vi "BarcodeFunc (1).vi"() -> ()   [LabVIEW 2016, in "Team234_Project5.lvrbt"]
uses:
  Team234_Project5.lvrbt
  <vilib>/NXT/Block Support/NXT_InputPort.ctl
  <vilib>/NXT/Subs/ColorSensorColors.ctl
  <vilib>/NXT/Subs/LVHSConnector.ctl
  <vilib>/NXT/LegoClasses/BrickReference/BrickReference.lvclass
  <vilib>/NXT/Block Support/NXT_OutputPort.ctl
  <vilib>/NXT/Dual Mode Library/Sensors/EV3_Color_Color.vi
  <vilib>/NXT/Dual Mode Library/Sound/Tone.vi
  <vilib>/NXT/NXTIO Xnodes/NXTIONodeSubVIs/NXTMoveMotors.vi
  <vilib>/NXT/Dual Mode Library/Waits/Wait_Num.vi
  <vilib>/NXT/NXTIO Xnodes/AddressXNode/NXTIOAddress.xnode
  <vilib>/NXT/NXTIO Xnodes/NXTIOXNode/NXTIO.xnode
panel:
  in  "NXT/EV3":T1
  out "NXT/EV3 10":T1
  in  "Time (1 sec) 3":sgl=1.0
  in  "Power/Speed 6":i8=75
  in  "Power/Speed 5":i8=75
  out "NXT/EV3 9":T1
  in  "Tone (440 Hz) 3":u16=440
  in  "Duration (500 ms) 3":u16=500
  out "Detected Color 2":T2
  in  "Port (Port 1) 2":T3 items=["Port 1", "Port 2", "Port 3", "Port 4"]
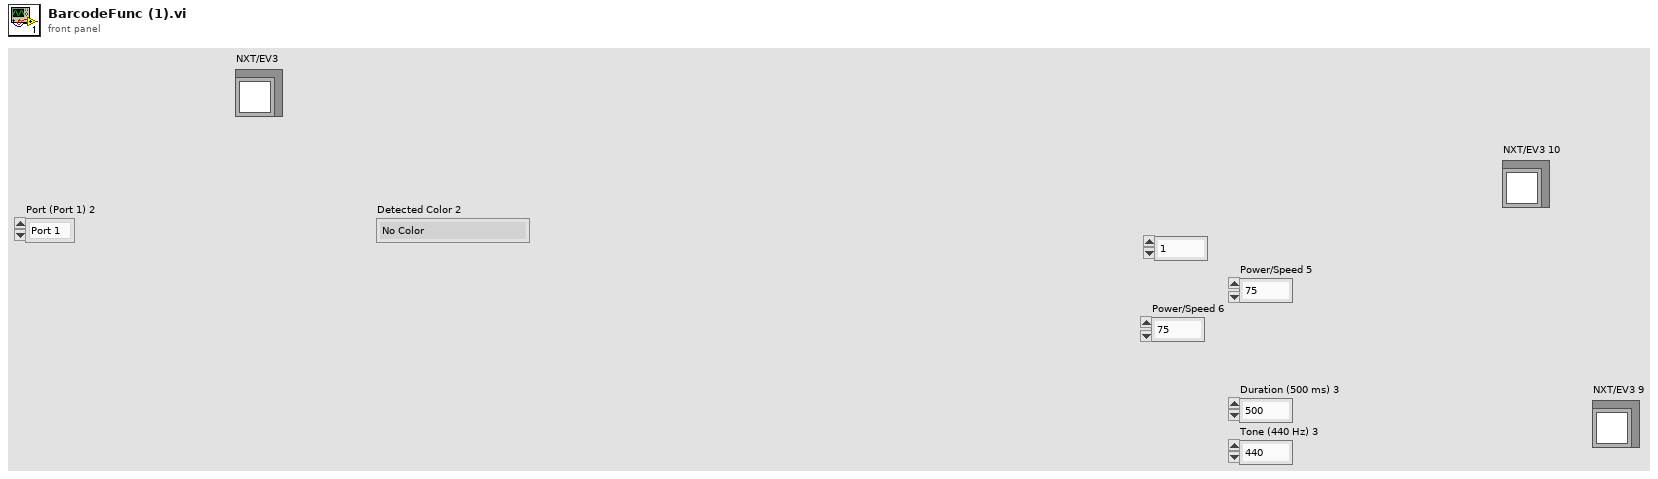
[diagram p1: front panel]
types:
  T1 = typedef "LVHSConnector.ctl" = refnum<class "BrickReference.lvclass">
  T2 = typedef "ColorSensorColors.ctl" = enum16{"No Color", "Black", "Blue", "Green", "Yellow", "Red", "White", "Brown"}
  T3 = typedef "NXT_InputPort.ctl" = u32
  T4 = typedef "NXT_OutputPort.ctl" = u8
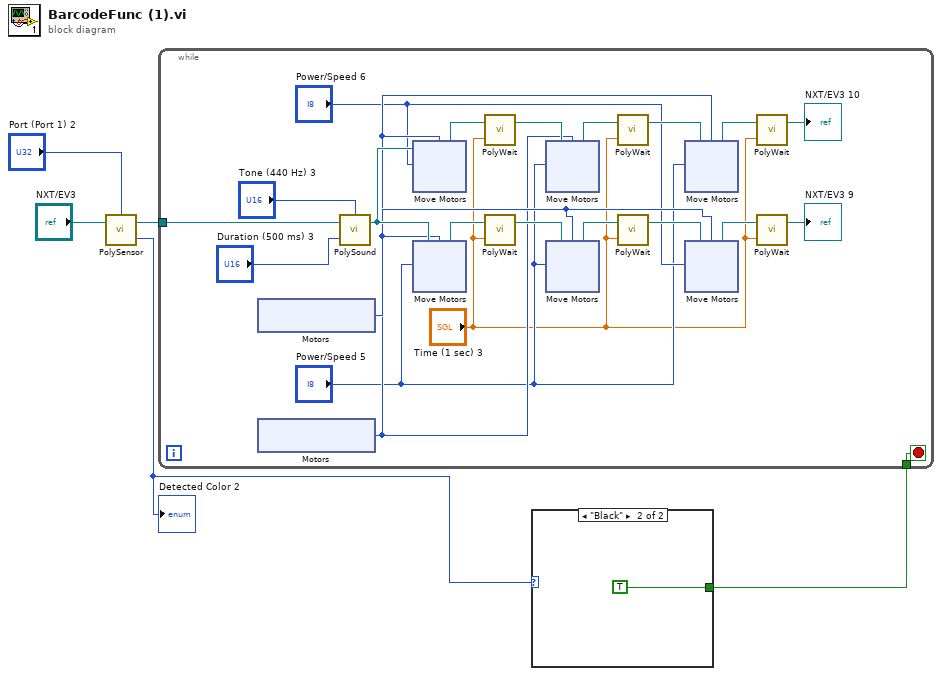
[diagram p0: block diagram]
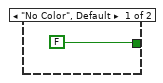
[diagram p2: hidden frame]
diagram:
  n1 = call-poly <vilib>:"PolySensor.vi"("NXT/EV3"="NXT/EV3", "Port (Port 1)"="Port (Port 1) 2") -> ("Detected Color"=w2:T2, "NXT/EV3"=w3:T1)  [unwired: 1 in]
  "Detected Color 2" <- w2
  n2 = case shown="\"Black\"" w2 {
    tunnel: [FALSE TRUE] -> w1
    frame "No Color", Default {
    }
    frame "Black" {
    }
  }
  n3 = while {
    tunnel: w3 -> [w9]
    tunnel: w1 -> [w8]
    stop <- w8 stop-if-true
    n4 = xnode "Motors"() -> ("Motor"=w18:T4)
    n5 = xnode "Motors"() -> ("Motor"=w17:T4)
    n6 = call-poly <vilib>:"PolySound.vi"("Duration (500 ms)"="Duration (500 ms) 3", "NXT/EV3"=w9, "Tone (440 Hz)"="Tone (440 Hz) 3") -> ("NXT/EV3"=w27:T1)  [unwired: 1 in]
    n7 = xnode "Move Motors"("Power/Speed 1"="Power/Speed 6", "Motors"=w17, "NXT/EV3"=w27) -> ("NXT/EV3"=w24:T1)
    n8 = xnode "Move Motors"("Power/Speed 1"="Power/Speed 5", "Motors"=w18, "NXT/EV3"=w27) -> ("NXT/EV3"=w26:T1)
    n9 = call-poly <vilib>:"PolyWait.vi"("Time (1 sec)"="Time (1 sec) 3", "NXT/EV3"=w24) -> ("NXT/EV3"=w23:T1)  [unwired: 2 in]
    n10 = call-poly <vilib>:"PolyWait.vi"("Time (1 sec)"="Time (1 sec) 3", "NXT/EV3"=w26) -> ("NXT/EV3"=w25:T1)  [unwired: 2 in]
    n11 = xnode "Move Motors"("Power/Speed 1"="Power/Speed 5", "Motors"=w17, "NXT/EV3"=w23) -> ("NXT/EV3"=w21:T1)
    n12 = xnode "Move Motors"("Power/Speed 1"="Power/Speed 5", "Motors"=w18, "NXT/EV3"=w25) -> ("NXT/EV3"=w22:T1)
    n13 = call-poly <vilib>:"PolyWait.vi"("Time (1 sec)"="Time (1 sec) 3", "NXT/EV3"=w21) -> ("NXT/EV3"=w19:T1)  [unwired: 2 in]
    n14 = call-poly <vilib>:"PolyWait.vi"("Time (1 sec)"="Time (1 sec) 3", "NXT/EV3"=w22) -> ("NXT/EV3"=w20:T1)  [unwired: 2 in]
    n15 = xnode "Move Motors"("Power/Speed 1"="Power/Speed 5", "Motors"=w17, "NXT/EV3"=w19) -> ("NXT/EV3"=w13:T1)
    n16 = xnode "Move Motors"("Power/Speed 1"="Power/Speed 6", "Motors"=w18, "NXT/EV3"=w20) -> ("NXT/EV3"=w14:T1)
    n17 = call-poly <vilib>:"PolyWait.vi"("Time (1 sec)"="Time (1 sec) 3", "NXT/EV3"=w13) -> ("NXT/EV3"=→"NXT/EV3 10":T1)  [unwired: 2 in]
    n18 = call-poly <vilib>:"PolyWait.vi"("Time (1 sec)"="Time (1 sec) 3", "NXT/EV3"=w14) -> ("NXT/EV3"=→"NXT/EV3 9":T1)  [unwired: 2 in]
  }
